vi "Simple Framework.vi"() -> ()   [LabVIEW 2014]
uses:
  IO Node Logic Template.lvlib
  <vilib>/SPIAPI/DIO/SPI Digital IO Lines.ctl
  <vilib>/SPIAPI/DIO/SPI DIO Enable Lines.ctl
  <userlib>/_NI SPI IP/FPGA/Controllers/Public/Spi Master Outputs.ctl
  <userlib>/_NI SPI IP/FPGA/Controllers/NI SPI IP (FPGA).lvlib
panel:
  in  "Command":T1
  out "spi output":T2
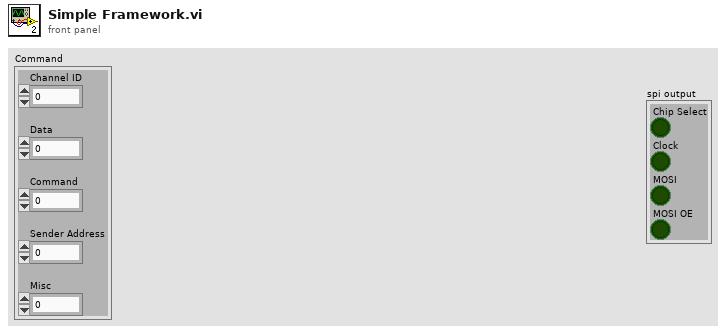
[diagram p1: front panel]
types:
  T1 = cluster{"Channel ID":u8, "Data":u64, "Command":u8, "Sender Address":u8, "Misc":u8}
  T2 = typedef "NI SPI IP (FPGA).lvlib/Spi Master Outputs.ctl" = cluster{"Chip Select":bool, "Clock":bool, "MOSI":bool, "MOSI OE":bool}
  T3 = typedef "SPI DIO Enable Lines.ctl" = cluster{"SCLK_en":refnum<k21>, "MISO_en":refnum<k21>, "MOSI_en":refnum<k21>, "CS0_en":refnum<k21>, "CS1_en":refnum<k21>, "CS2_en":refnum<k21>, "CS3_en":refnum<k21>, "CS4_en":refnum<k21>, "CS5_en":refnum<k21>}
  T4 = typedef "SPI Digital IO Lines.ctl" = cluster{"SCLK":refnum<k21>, "MISO":refnum<k21>, "MOSI":refnum<k21>, "CS 0":refnum<k21>, "CS 1":refnum<k21>, "CS 2":refnum<k21>, "CS 3":refnum<k21>, "CS 4":refnum<k21>, "CS 5":refnum<k21>}
  T5 = typedef "IO Node Logic Template.lvlib/All Nodes Resources.ctl" = cluster{"FIFOs.Node 0":T6}
  T6 = typedef "IO Node Logic Template.lvlib/NodeResources FIFOs.ctl" = cluster{"SendCmdFIFO":refnum<k21>, "ReceiveDataFIFO":refnum<k21>}
  T7 = typedef "Internal Data (SPI API).ctl" = cluster{"DLU To SPI Engine Data FIFO":refnum<k21>, "SPI Engine to DLU Data FIFO":refnum<k21>, "Data to SPI Engine (Cache) Register":refnum<k21>, "SPI PHY Settings to SPI Engine (Cahche) Register":refnum<k21>}
  T8 = typedef "NI SPI IP (FPGA).lvlib/Spi Master Inputs.ctl" = cluster{"MISO":bool}
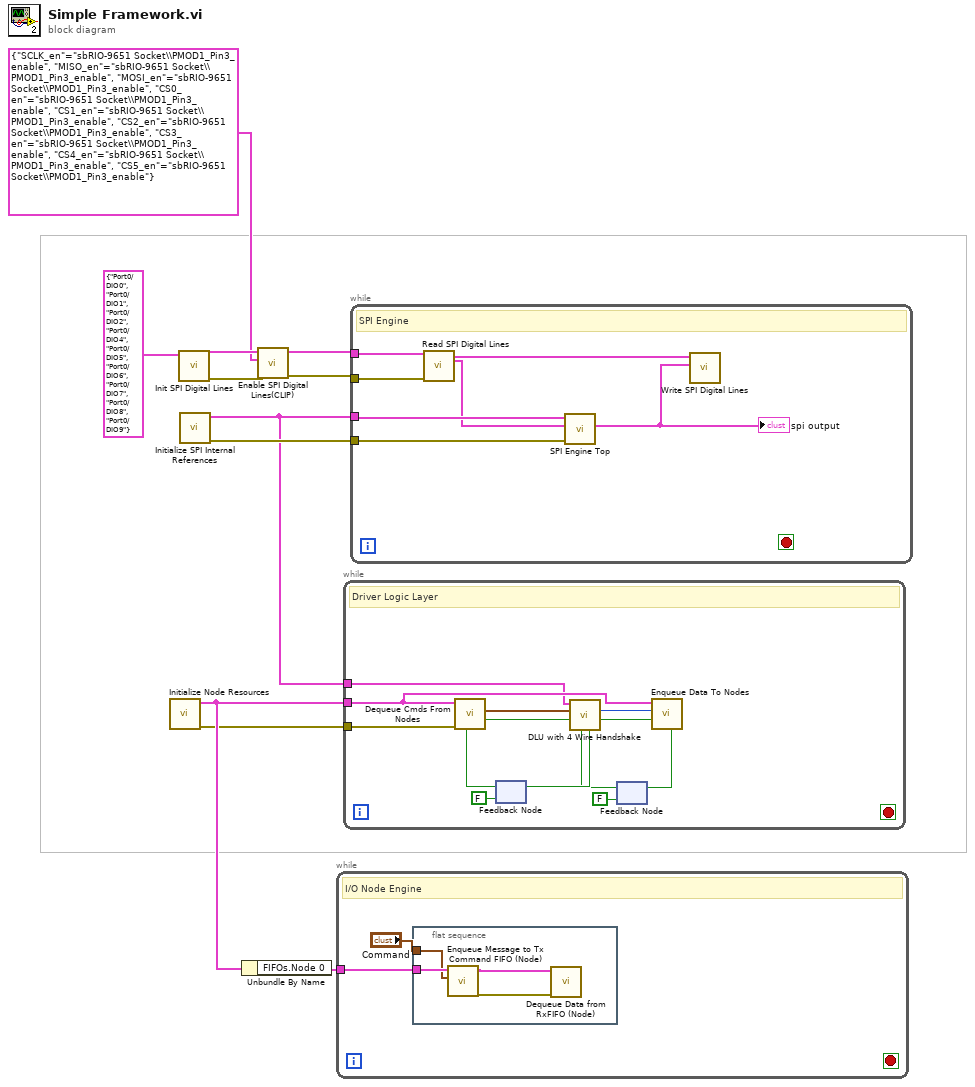
[diagram p0: block diagram]
diagram:
  n1 = call "Initialize Node Resources.vi"() -> ("error out"=w9:errorcluster, "Communication FIFOs"=w10:T5)  [unwired: 10 in]
  n2 = call <vilib>:"Init SPI Digital Lines.vi"("Chip Select DIO Lines"=T4 {"SCLK"="Port0/DIO0", "MISO"="Port0/DIO1", "MOSI"="Port0/DIO2", "CS 0"="Port0/DIO4", "CS 1"="Port0/DIO5", "CS 2"="Port0/DIO6", "CS 3"="Port0/DIO7", "CS 4"="Port0/DIO8", "CS 5"="Port0/DIO9"}) -> ("error out"=w4:errorcluster, "Chip Select DIO Lines"=w5:T4)  [unwired: 9 in]
  n3 = call <vilib>:"Initialize SPI Internal References.vi"() -> ("error out"=w8:errorcluster, "SPI API References"=w7:T7)  [unwired: 10 in]
  n4 = Unbundle By Name(w10) -> ("FIFOs.Node 0"=w11:T6)
  n5 = call <vilib>:"Enable SPI Digital Lines(CLIP).vi"("error in"=w4, "Enable Lines"=T3 {"SCLK_en"="sbRIO-9651 Socket\\PMOD1_Pin3_enable", "MISO_en"="sbRIO-9651 Socket\\PMOD1_Pin3_enable", "MOSI_en"="sbRIO-9651 Socket\\PMOD1_Pin3_enable", "CS0_en"="sbRIO-9651 Socket\\PMOD1_Pin3_enable", "CS1_en"="sbRIO-9651 Socket\\PMOD1_Pin3_enable", "CS2_en"="sbRIO-9651 Socket\\PMOD1_Pin3_enable", "CS3_en"="sbRIO-9651 Socket\\PMOD1_Pin3_enable", "CS4_en"="sbRIO-9651 Socket\\PMOD1_Pin3_enable", "CS5_en"="sbRIO-9651 Socket\\PMOD1_Pin3_enable"}, "SPI DIO Lines"=w5) -> ("error out"=w3:errorcluster, "Chip Select DIO Lines"=w2:T4)  [unwired: 7 in]
  n6 = while {
    tunnel: w11 -> [w13]
    stop <- _ stop-if-true
    # "I/O Node Engine"
    n7 = flat-sequence {
      tunnel: w13 -> [w16]
      tunnel: "Command" -> [w14]
      frame #0 {
        n8 = call "Enqueue Message to Tx Command FIFO (Node).vi"("Command"=w14, "FIFOs: I/O Node"=w16) -> ("error out"=w17:errorcluster, "FIFOs: I/O Node"=w15:T6)  [unwired: 7 in, 1 out]
        n9 = call "Dequeue Data from RxFIFO (Node).vi"("error in"=w17, "FIFOs: I/O Node"=w15) -> ()  [unwired: 6 in, 4 out]
      }
    }
  }
  n10 = while {
    tunnel: w10 -> [w19]
    tunnel: w9 -> [w20]
    tunnel: w7 -> [w18]
    stop <- _ stop-if-true
    # "Driver Logic Layer"
    n11 = feedback #1(FALSE ("Ready For Input?")) -> (w27:bool)
    n12 = call "Dequeue Cmds From Nodes.vi"("Ready For Output?"=w27, "error in"=w20, "Communication FIFOs"=w19) -> ("Cmd Received Valid"=w25:bool, "Cmd Received"=w24:T1)  [unwired: 5 in, 2 out]
    n13 = feedback #2(FALSE ("Ready for Input")) -> (w22:bool)
    n14 = call "DLU with 4 Wire Handshake.vi"("ready for output"=w22, "Input Valid"=w25, "Input Data"=w24, "Private Data In"=w18) -> ("Output Valid"=w30:bool, "Output Data"=w29:u64, "ready for Input"=w26:bool)  [unwired: 5 in]
    n15 = feedback-in #1(w26) -> ()
    n16 = call "Enqueue Data To Nodes.vi"("Input Valid"=w30, "Input Data"=w29, "Communication FIFOs"=w19) -> ("Ready for Input"=w23:bool)  [unwired: 7 in, 1 out]
    n17 = feedback-in #2(w23) -> ()
  }
  n18 = while {
    tunnel: w7 -> [w37]
    tunnel: w8 -> [w36]
    tunnel: w2 -> [w35]
    tunnel: w3 -> [w34]
    stop <- _ stop-if-true
    # "SPI Engine"
    n19 = call <vilib>:"Read SPI Digital Lines.vi"("Chip Select DIO Lines"=w35, "error in"=w34) -> ("Chip Select DIO Lines Out"=w33:T4, "SPI Read Data"=w31:T8)  [unwired: 11 in, 1 out]
    n20 = call <vilib>:"SPI Engine Top.vi"("error in"=w36, "SPI Read Data"=w31, "SPI API References"=w37) -> ("SPI DIO Output"=w32:T2)  [unwired: 6 in, 2 out]
    "spi output" <- w32
    n21 = call <vilib>:"Write SPI Digital Lines.vi"("spi output"=w32, "Chip Select DIO Lines"=w33) -> ()  [unwired: 8 in, 2 out]
  }
